vi "Config Type.vi"(11 "SeqRunning Condition in":refnum<class "SeqRunning Condition.lvclass">) -> (2 "Condition Config":refnum<class "Condition Config.lvclass">)   [LabVIEW 2020, in "VolatusSeq.lvlib" / "SeqRunning Condition.lvclass"]
uses:
  SeqRunning Condition.lvclass
  SeqRunning Condition.lvclass/SeqRunning Condition.ctl
  VolatusSeqConfig/SeqRunning Condition Config/SeqRunning Condition Config.lvclass
  C:/dev/lv20CE/relink/lv-volatus/VolatusSeqConfig/Condition Config/Condition Config.lvclass
  C:/dev/lv20CE/relink/lv-volatus/VolatusSeqConfig/SeqRunning Condition Config/SeqRunning Condition Config.lvclass
  VolatusSeqConfig/Condition Config/Condition Config.lvclass
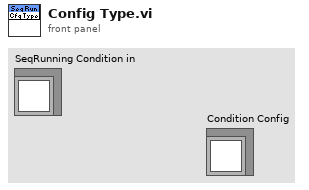
[diagram p1: front panel]
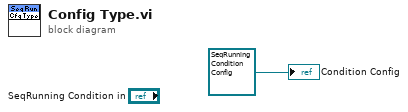
[diagram p0: block diagram]
diagram:
  "Condition Config" <- refnum<class "SeqRunning Condition Config.lvclass"> refnum ("VolatusSeqConfig.lvlib:SeqRunning Condition Config.lvclass")
